vi "HostFPGAMonitor.vi"() -> ()   [LabVIEW 2014]
uses:
  <vilib>/userdefined/High Color/nirio_resource_hc.ctl
  <vilib>/FPGAPlugInAG/PCIe-7851R/niLvFpga_Open_PCIe-7851R.vi
  <vilib>/rvi/interface/common/dynamic/niFpgaDynamicAddResources.vi
  <vilib>/Utility/error.llb/Error Cluster From Error Code.vi
  <vilib>/rvi/errors/niLvFpgaAdjustHostInterfaceError.vi
  <vilib>/FPGAPlugInAG/Dynamic/niLvFpga_Close_Dynamic.vi
  <vilib>/rvi/interface/nirviOpenFPGA/nirviOpenFPGA.xnode
  FPGA Bitfiles/UntitledProject1_FPGATarget_FPGAHoppingSimul_0VGbdY9yR1g.lvbitx
  <vilib>/rvi/interface/nirviReadWriteControl/nirviReadWriteControl.xnode
  <vilib>/rvi/interface/nirviMethod/nirviMethod.xnode
  <vilib>/rvi/interface/nirviCloseFPGA/nirviCloseFPGA.xnode
  <vilib>/rvi/interface/Simulation/niFpgaSimulationCallBeginRW.vi
  NiFpgaLv.dll
  <vilib>/FPGAPlugInAG/Dynamic/niLvFpga_ReadFifo_Dynamic.vi
  <vilib>/rvi/errors/niLvFpgaMergeErrorWithErrorCode.vi
panel:
  out "TimeDelta":u32
  out "WriteNum":u32
  out "Waveform Chart":i16(graph)
  in  "stop":bool
  in  "Sleep":u32
  in  "BaseTime us":i16
  in  "PIZ":T1
  in  "Counting":i32
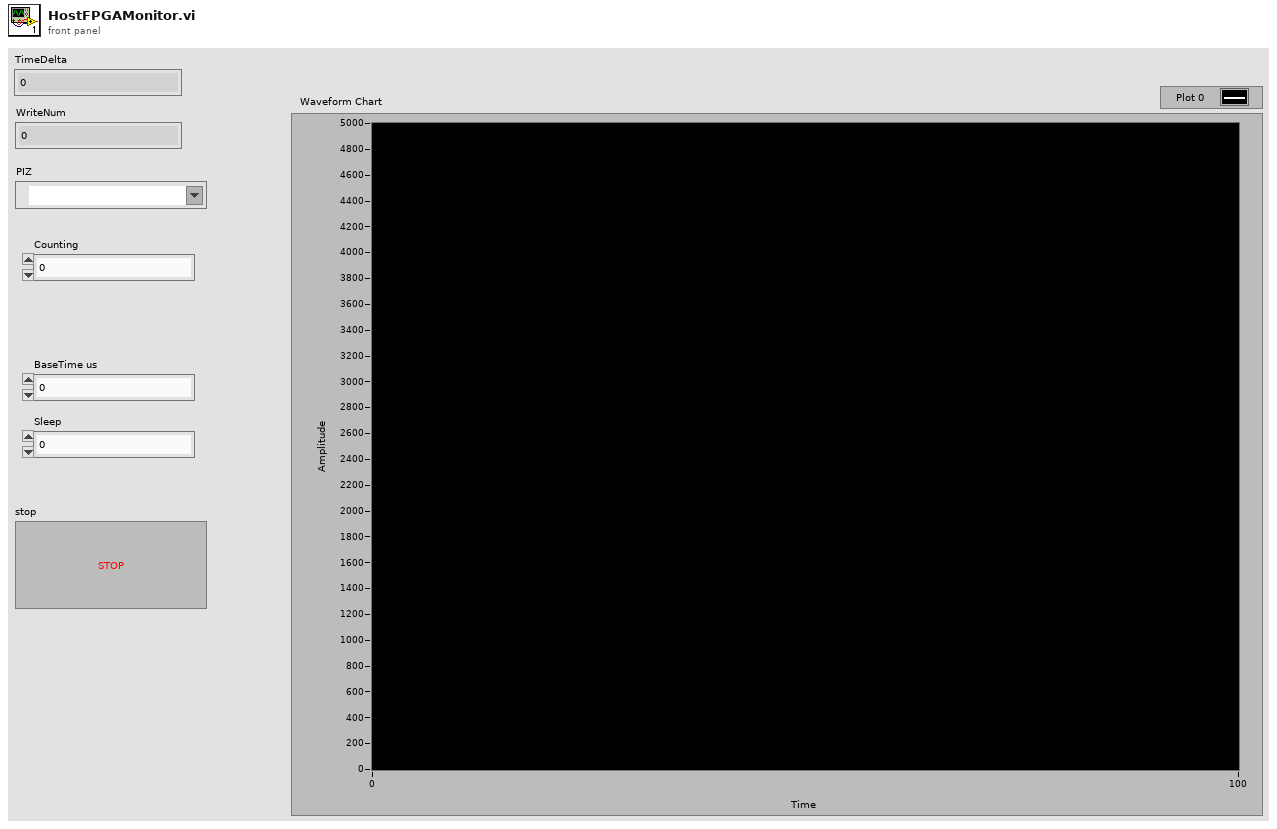
[diagram p1: front panel]
types:
  T1 = typedef "nirio_resource_hc.ctl" = tag
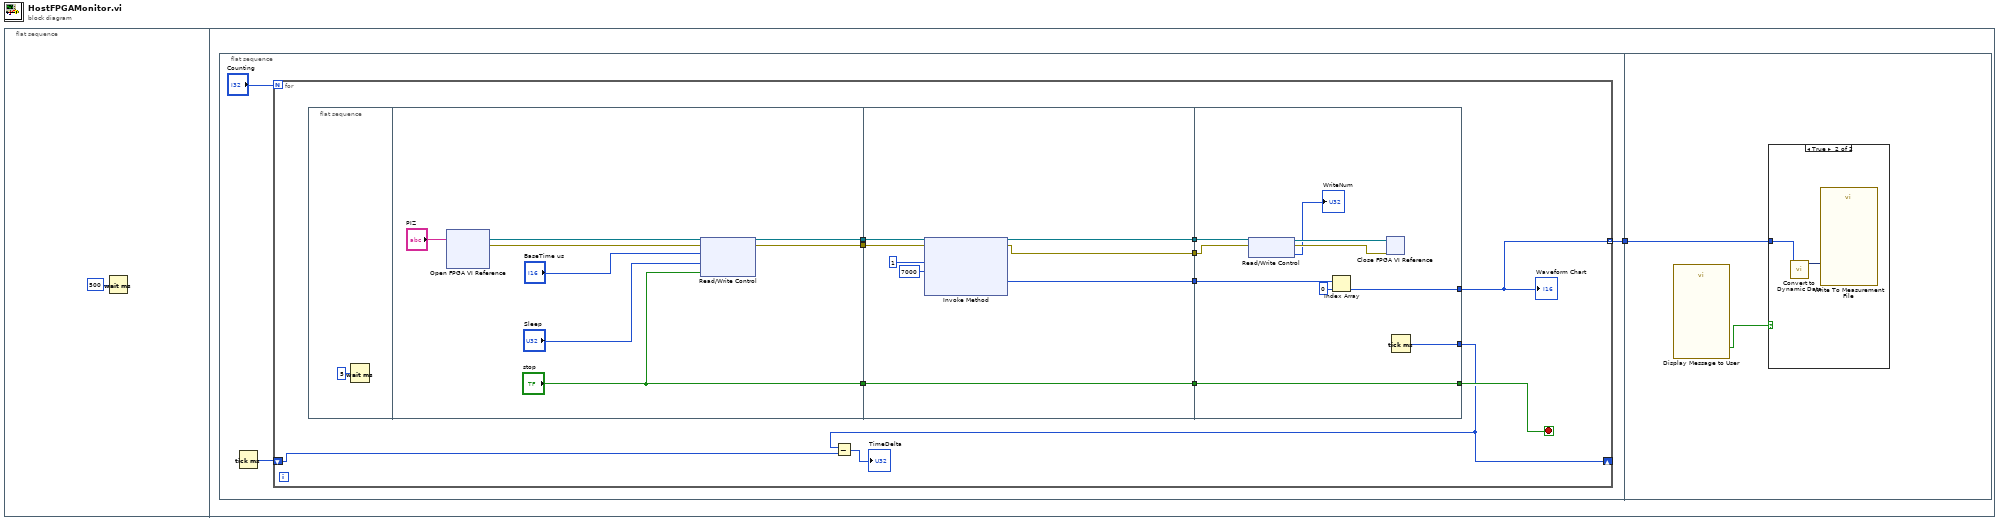
[diagram p0: block diagram]
diagram:
  n1 = flat-sequence {
    frame #0 {
      n2 = Wait (ms)(milliseconds to wait=u32 500) -> ()  [unwired: 1 out]
    }
    frame #1 {
      n3 = flat-sequence {
        tunnel: [w4] -> w2
        tunnel: w2 -> [w45]
        frame #0 {
          n4 = Tick Count (ms)() -> (millisecond timer value=w3:u32)
          n5 = for {
            N: "Counting" -> [_]
            tunnel: [w9] -> w4 mode=indexing
            shift-right: [w7] -> _
            shift-left: w3 -> [w6]
            stop <- w17 stop-if-true
            n6 = flat-sequence {
              tunnel: ["stop"] -> w15
              tunnel: [w20] -> w14
              tunnel: [w19] -> w13
              tunnel: [w34] -> w16
              tunnel: w15 -> [w34]
              tunnel: w14 -> [w33]
              tunnel: w13 -> [w32]
              tunnel: [w31] -> w12
              tunnel: [w30] -> w11
              tunnel: [w29] -> w10
              tunnel: [w44] -> w17
              tunnel: w16 -> [w44]
              tunnel: w12 -> [w43]
              tunnel: w11 -> [w40]
              tunnel: w10 -> [w39]
              tunnel: [w41] -> w9
              tunnel: [w35] -> w7
              frame #0 {
                n7 = Wait (ms)(milliseconds to wait=u32 5) -> ()  [unwired: 1 out]
              }
              frame #1 {
                n8 = xnode "Open FPGA VI Reference"("resource name"="PIZ") -> ("FPGA VI Reference Out"=w25:refnum<k20>, "error out"=w24:errorcluster)  [unwired: 1 in]
                n9 = xnode "Read/Write Control"("FPGA VI Reference In"=w25, "error in"=w24, "BaseTime us"="BaseTime us", "Sleep"="Sleep", "stop"="stop") -> ("FPGA VI Reference Out"=w20:refnum<k20>, "error out"=w19:errorcluster)
              }
              frame #2 {
                n10 = xnode "Invoke Method"("FPGA VI Reference In"=w33, "error in"=w32, "Number of Elements"=u32 1, "Timeout (ms)"=7000) -> ("FPGA VI Reference Out"=w30:refnum<k20>, "error out"=w29:errorcluster, "Data"=w31:i16[])  [unwired: 1 out]
              }
              frame #3 {
                n11 = xnode "Read/Write Control"("FPGA VI Reference In"=w40, "error in"=w39) -> ("FPGA VI Reference Out"=w38:refnum<k20>, "error out"=w37:errorcluster, "WriteNum"=→"WriteNum":u32)
                n12 = Index Array(array=w43, index=0) -> (element=w41:i16)
                n13 = xnode "Close FPGA VI Reference"("FPGA VI Reference In"=w38, "error in"=w37) -> ()  [unwired: 1 out]
                n14 = Tick Count (ms)() -> (millisecond timer value=w35:u32)
              }
            }
            n15 = Subtract(x=w7, y=w6) -> (x-y=→"TimeDelta":u32)
            "Waveform Chart" <- w9
          }
        }
        frame #1 {
          n16 = call "Display Message to User"() -> ("OK"=w46:bool)  [unwired: 10 in, 1 out]
          n17 = case shown="True" w46 {
            tunnel: w45 -> [_ w48]
            frame False {
            }
            frame True {
              n18 = call "Convert to Dynamic Data"("Array"=w48) -> ("Dynamic Data Type"=w47:dynamicdata)  [unwired: 3 in]
              n19 = call "Write To Measurement File"("Signals"=w47) -> ()  [unwired: 16 in, 3 out]
            }
          }
        }
      }
    }
  }
